vi "Are_Items_Visible_Files.vi"(8 "error in (no error)":errorcluster, 11 "AB_Dest_App in":refnum<class "AB_Dest_App.lvclass">) -> (0 "error out":errorcluster, 2 "itemsVisibleFiles":bool, 3 "AB_Dest_App out":refnum<class "AB_Dest_App.lvclass">)   [LabVIEW 2020, in "AB_Dest_App.lvclass"]
uses:
  <vilib>/AppBuilder/AB_Classes/Destination/Dest_Application/AB_Dest_App.lvclass
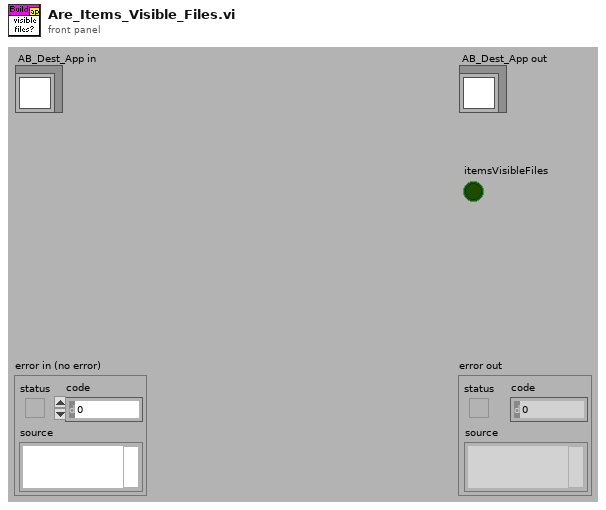
[diagram p1: front panel]
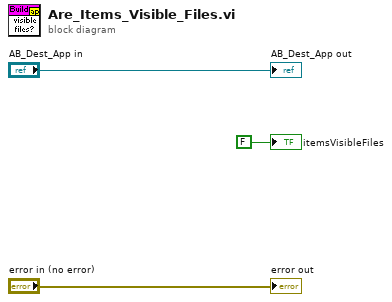
[diagram p0: block diagram]
diagram:
  "error out" <- "error in (no error)"
  "AB_Dest_App out" <- "AB_Dest_App in"
  "itemsVisibleFiles" <- FALSE ("itemsVisibleFiles")
